vi "getConnectionPoint.vi"(0 "reference":refnum<class "InitialStateNode.lvclass">, 1 "direction":refnum<class "Direction.lvclass">, 5 "error in (no error)":errorcluster) -> (14 "reference out":refnum<class "InitialStateNode.lvclass">, 15 "point2D":T1 {"y" format="%.2f"; "x" format="%.2f"}, 19 "error out":errorcluster)   [LabVIEW 2014, in "InitialStateNode.lvclass"]
doc: "getConnectionPoint"
uses:
  <resource>/Framework/Providers/Open_GDS/UML/InitialStateNode_class/InitialStateNode.lvclass
  <resource>/Framework/Providers/Open_GDS/UML/Direction_class/Direction.lvclass
  <resource>/Framework/Providers/Open_GDS/UML/General/Point/Point Point2D.ctl
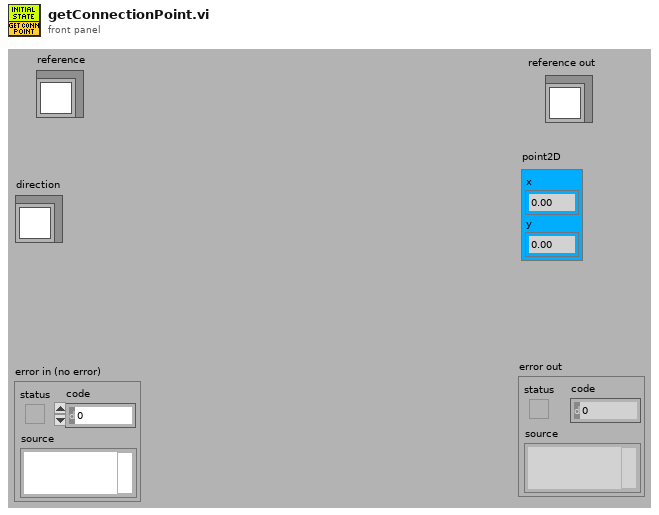
[diagram p1: front panel]
types:
  T1 = typedef "Point Point2D.ctl" = cluster{"x":dbl, "y":dbl}
  T2 = typedef "InitialStateNode.lvclass/ObjectAttributes.ctl" = cluster{"Base class":T3, "name":refnum<class "MultiLineString.lvclass">, "DEFAULT_WIDTH":i32, "DEFAULT_HEIGHT":i32}
  T3 = typedef "RectangularNode.lvclass/ObjectAttributes.ctl" = cluster{"Base class":T4, "bounds":T5}
  T4 = typedef "AbstractNode.lvclass/ObjectAttributes.ctl" = cluster{"parent":refnum<class "AbstractNode.lvclass">, "children":refnum<class "AbstractNode.lvclass">[], "Hidden":bool}
  T5 = typedef "Rectangle Rectangle2D.ctl" = cluster{"x":dbl, "y":dbl, "width":dbl, "height":dbl}
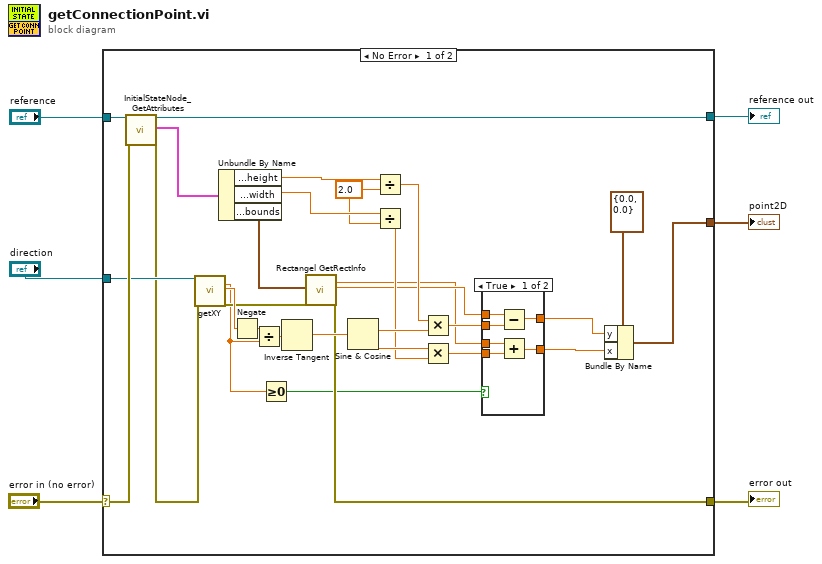
[diagram p0: block diagram]
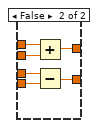
[diagram p2: hidden frame]
diagram:
  n1 = case shown="No Error" "error in (no error)" {
    selector: "error in (no error)" -> [w36 w49]
    tunnel: "reference" -> [w35 w50]
    tunnel: [w10 w49] -> w4
    tunnel: [w34 w50] -> w3
    tunnel: "direction" -> [w31 _]
    tunnel: [w11 _] -> w1
    frame No Error {
      w26 = 2.0 ("y")
      n2 = call <resource>:"InitialStateNode_GetAttributes.vi"("reference in"=w35, "error in (no error)"=w36) -> ("reference out"=w34:refnum<class "InitialStateNode.lvclass">, "Attributes"=w32:T2, "error out"=w30:errorcluster)  [unwired: 15 out]
      n3 = call <resource>:"getXY.vi"("reference"=w31, "error in (no error)"=w30) -> ("x"=w8:dbl, "y"=w33:dbl, "error out"=w25:errorcluster)  [unwired: 15 out]
      n4 = Unbundle By Name(w32) -> ("Base class.bounds.height"=w28:dbl, "Base class.bounds.width"=w27:dbl, "Base class.bounds"=w24:T5)
      n5 = Negate(x=w33) -> (-x=w9:dbl)
      n6 = Divide(x=w9, y=w8) -> (x/y=w29:dbl)
      n7 = Greater Or Equal To 0?(x=w8) -> (x >= 0?=w7:bool)
      n8 = Inverse Tangent(1:w29) -> (0:w23:dbl)
      n9 = call <resource>:"Rectangel GetRectInfo.vi"("bounds"=w24, "error in (no error)"=w25) -> ("centerX"=w15:dbl, "centerY"=w16:dbl, "error out"=w10:errorcluster)  [unwired: 15 out]
      n10 = Sine & Cosine(0:w23) -> (1:w21:dbl, 2:w22:dbl)
      n11 = Divide(x=w28, y=w26) -> (x/y=w20:dbl)
      n12 = Divide(x=w27, y=w26) -> (x/y=w19:dbl)
      n13 = Multiply(x=w20, y=w21) -> (x*y=w18:dbl)
      n14 = Multiply(x=w22, y=w19) -> (x*y=w17:dbl)
      n15 = case shown="True" w7 {
        tunnel: w18 -> [w42 w48]
        tunnel: w17 -> [w41 w47]
        tunnel: w16 -> [w40 w46]
        tunnel: w15 -> [w39 w45]
        tunnel: [w38 w44] -> w13
        tunnel: [w37 w43] -> w12
        frame True {
          n16 = Subtract(x=w40, y=w42) -> (x-y=w38:dbl)
          n17 = Add(x=w39, y=w41) -> (x+y=w37:dbl)
        }
        frame False {
          n18 = Add(x=w46, y=w48) -> (x+y=w44:dbl)
          n19 = Subtract(x=w45, y=w47) -> (x-y=w43:dbl)
        }
      }
      n20 = Bundle By Name(cluster=T1 {"x"=0.0, "y"=0.0} ("point2D"), "y"=w13, "x"=w12) -> (w11:T1)
    }
    frame Error {
    }
  }
  "reference out" <- w3
  "error out" <- w4
  "point2D" <- w1
